vi "side_zeta_microstep.vi"(0 "Zeta_B":i32, 1 "Step":i32, 2 "Zeta_F":i32, 3 "taget_f":i32, 4 "Delay":i32, 5 "target_b":i32) -> (6 "OZeta_b":i32, 7 "Done":bool, 8 "Ozeta_f":i32)   [LabVIEW 2017]
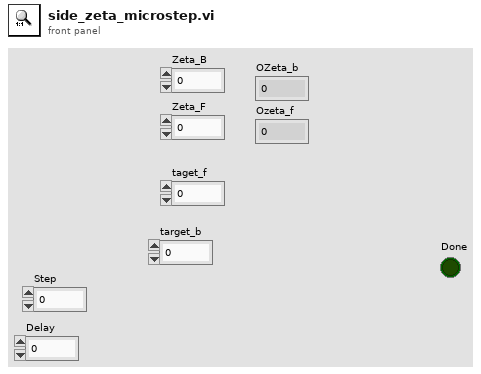
[diagram p1: front panel]
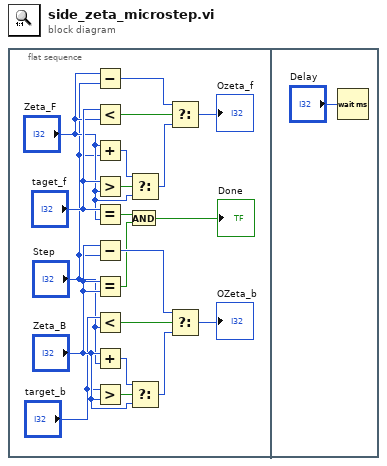
[diagram p0: block diagram]
diagram:
  n1 = flat-sequence {
    frame #0 {
      n2 = Subtract(x="Zeta_F", y="Step") -> (x-y=w12:i32)
      n3 = Less?(x="taget_f", y="Zeta_F") -> (x < y?=w14:bool)
      n4 = Add(x="Zeta_F", y="Step") -> (x+y=w20:i32)
      n5 = Greater?(x="taget_f", y="Zeta_F") -> (0:w18:bool)
      n6 = Equal?(x="taget_f", y="Zeta_F") -> (x = y?=w7:bool)
      n7 = Subtract(x="Zeta_B", y="Step") -> (x-y=w11:i32)
      n8 = Equal?(x="Zeta_B", y="Zeta_B") -> (x = y?=w6:bool)
      n9 = Less?(x="target_b", y="Step") -> (x < y?=w13:bool)
      n10 = Add(x="Zeta_B", y="Step") -> (x+y=w19:i32)
      n11 = Greater?(x="target_b", y="Zeta_B") -> (0:w17:bool)
      n12 = And(x=w7, y=w6) -> (x .and. y?=→"Done":bool)
      n13 = Select(t=w20, s=w18, f="Zeta_F") -> (s? t:f=w15:i32)
      n14 = Select(t=w19, s=w17, f="Zeta_B") -> (s? t:f=w16:i32)
      n15 = Select(t=w12, s=w14, f=w15) -> (s? t:f=→"Ozeta_f":i32)
      n16 = Select(t=w11, s=w13, f=w16) -> (s? t:f=→"OZeta_b":i32)
    }
    frame #1 {
      n17 = Wait (ms)(milliseconds to wait="Delay") -> ()  [unwired: 1 out]
    }
  }
